vi "EE_PathToEdk.dll_Write.vi"(8 "error in (no error)":errorcluster, 10 "PathToEdk.dll":path=path "C:/Program Files/Emotiv Development Kit_v1.0.0.3-PREMIUM/edk.dll", 11 "EmotivEpocHeadsetControls in":refnum<class "EmotivEpocHeadsetControls.lvclass">) -> (0 "error out":errorcluster, 3 "EmotivEpocHeadsetControls out":refnum<class "EmotivEpocHeadsetControls.lvclass">)   [LabVIEW 2016, in "Emotiv Epoc.lvlib" / "EmotivEpocHeadsetControls.lvclass"]
uses:
  EmotivEpocHeadsetControls.lvclass
  EmotivEpocHeadsetControls.lvclass/EmotivEpocHeadsetControls.ctl
panel:
  # "This VI is a part of BCI Design library, http://www.ru-bci.org \nCopyright © 2020, Sotnikov Peter, All rights reserved. License: GNU GPLv3"
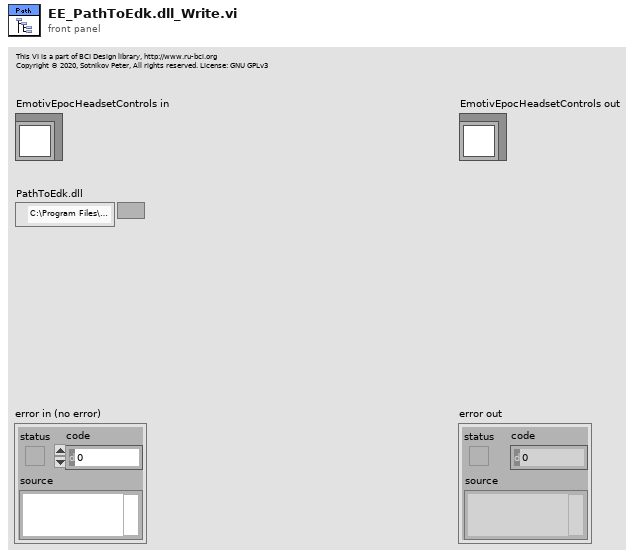
[diagram p1: front panel]
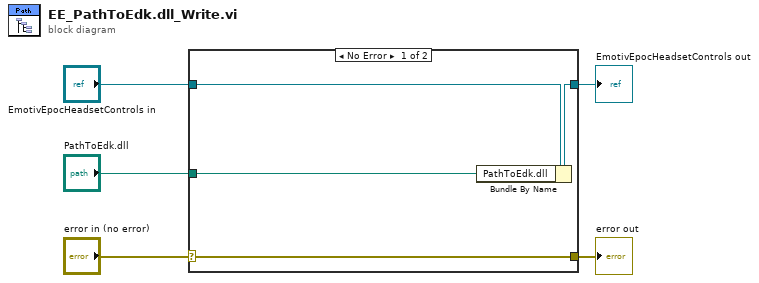
[diagram p0: block diagram]
diagram:
  n1 = case shown="No Error" "error in (no error)" {
    selector: "error in (no error)" -> [w9 w10]
    tunnel: [w9 w10] -> w4
    tunnel: [w7 w11] -> w2
    tunnel: "EmotivEpocHeadsetControls in" -> [w8 w11]
    tunnel: "PathToEdk.dll" -> [w6 _]
    frame No Error {
      n2 = Bundle By Name(cluster=w8, "PathToEdk.dll"=w6) -> (w7:refnum<class "EmotivEpocHeadsetControls.lvclass">)
    }
    frame Error {
    }
  }
  "error out" <- w4
  "EmotivEpocHeadsetControls out" <- w2
